vi "Cache.vi"(7 "Action":T1, 8 "error in (no error)":errorcluster, 10 "VI in":variant, 11 "Thread Name":string) -> (0 "error out":errorcluster, 1 "Found?":bool, 2 "VI out":variant, 3 "Generic VI out":refnum<vi>, 5 "Thread Names":string[](array[string]))   [LabVIEW 2018, in "Thread.lvlib"]
uses:
  Thread.lvlib
  Cache Action.ctl
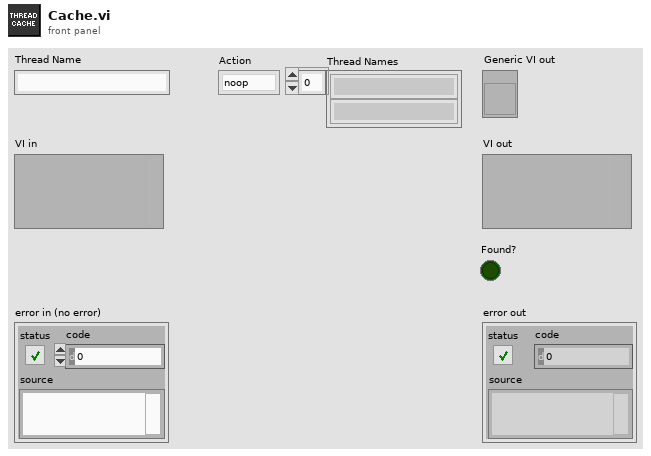
[diagram p1: front panel]
types:
  T1 = typedef "Thread.lvlib/Cache Action.ctl" = enum8{"noop", "get", "add", "remove", "remove_by_ref"}
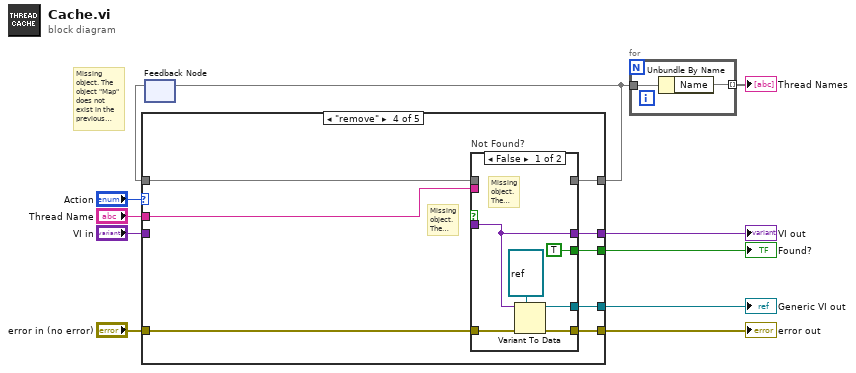
[diagram p0: block diagram]
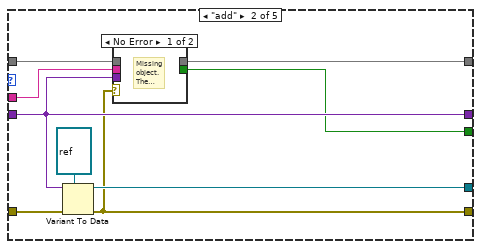
[diagram p3: hidden frame]
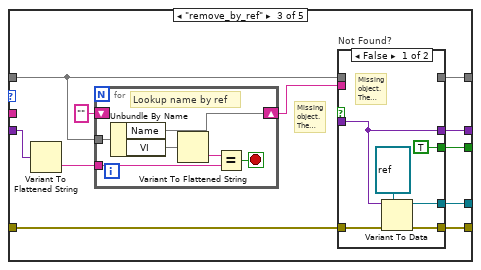
[diagram p5: hidden frame]
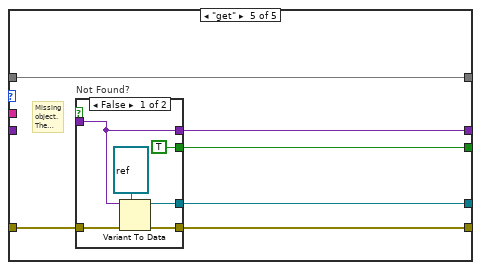
[diagram p8: hidden frame]
diagram:
  # "Missing object. The object \"Map\" does not exist in the previous version."
  n1 = feedback #1() -> (w8, w12)
  n2 = case shown="\"remove\"" "Action" {
    tunnel: [w13 w15 w34 w57 w72] -> w9
    tunnel: "error in (no error)" -> [w13 w23 w35 w58 w73]
    tunnel: [w14 w21 w32 w55 w68] -> w3
    tunnel: w8 -> [w14 w22 w28 w52 w68]
    tunnel: "Thread Name" -> [_ w20 _ w51 _]
    tunnel: "VI in" -> [_ w19 w29 _ _]
    tunnel: [_ w19 w31 w54 w70] -> w5
    tunnel: [_ w17 w33 w56 w71] -> w4
    tunnel: [_ w16 w30 w53 w69] -> w1
    frame "noop" {
    }
    frame "add" {
      n3 = Variant To Data(error in=w23, type=refnum<vi> refnum ("Generic VI out"), Variant=w19) -> (data=w17:refnum<vi>, error out=w15:errorcluster)
      n4 = case shown="No Error" w15 {
        tunnel: w22 -> [_ w24]
        tunnel: [_ w24] -> w21
        tunnel: w20 -> [_ _]
        tunnel: w19 -> [_ _]
        tunnel: [_ _] -> w16
        frame No Error {
          # "Missing object. The object \"Insert Into Map\" does not exist in the previous version."
        }
        frame Error {
        }
      }
    }
    frame "remove_by_ref" {
      # "Missing object. The object \"Look In Map\" does not exist in the previous version."
      n5 = Variant To Flattened String(Variant=w29) -> (data string=w26:string)  [unwired: 1 out]
      n6 = for {
        tunnel: w28 -> [w41]
        shift-right: [w39] -> w25
        shift-left: "" ("Name") -> [_]
        tunnel: w26 -> [w37]
        stop <- w36 stop-if-true
        # "Lookup name by ref"
        n7 = Unbundle By Name(w41) -> ("Name"=w39, "VI"=w40)
        n8 = Variant To Flattened String(Variant=w40) -> (data string=w38:string)  [unwired: 1 out]
        n9 = Equal?(x=w38, y=w37) -> (x = y?=w36:bool)
      }
      n10 = case "Not Found?" shown="False" {
        selector: _ -> [_ _]
        tunnel: w35 -> [w48 w49]
        tunnel: [w47 w49] -> w34
        tunnel: [w45 _] -> w33
        tunnel: w28 -> [_ w50]
        tunnel: [w44 w50] -> w32
        tunnel: w25 -> [_ _]
        tunnel: _ -> [w43 _]
        tunnel: [w43 _] -> w31
        tunnel: [TRUE _] -> w30
        frame False {
          # "Missing object. The object \"Remove From Map\" does not exist in the previous version."
          n11 = Variant To Data(error in=w48, type=refnum<vi> refnum ("Generic VI out"), Variant=w43) -> (data=w45:refnum<vi>, error out=w47:errorcluster)
        }
        frame True {
        }
      }
    }
    frame "remove" {
      # "Missing object. The object \"Look In Map\" does not exist in the previous version."
      n12 = case "Not Found?" shown="False" {
        selector: _ -> [_ _]
        tunnel: w58 -> [w65 w66]
        tunnel: [w64 w66] -> w57
        tunnel: [w62 _] -> w56
        tunnel: w52 -> [_ w67]
        tunnel: [w61 w67] -> w55
        tunnel: w51 -> [_ _]
        tunnel: _ -> [w60 _]
        tunnel: [w60 _] -> w54
        tunnel: [TRUE _] -> w53
        frame False {
          # "Missing object. The object \"Remove From Map\" does not exist in the previous version."
          n13 = Variant To Data(error in=w65, type=refnum<vi> refnum ("Generic VI out"), Variant=w60) -> (data=w62:refnum<vi>, error out=w64:errorcluster)
        }
        frame True {
        }
      }
    }
    frame "get" {
      # "Missing object. The object \"Look In Map\" does not exist in the previous version."
      n14 = case "Not Found?" shown="False" {
        selector: _ -> [_ _]
        tunnel: w73 -> [w79 w80]
        tunnel: [w78 w80] -> w72
        tunnel: [w76 _] -> w71
        tunnel: _ -> [w75 _]
        tunnel: [w75 _] -> w70
        tunnel: [TRUE _] -> w69
        frame False {
          n15 = Variant To Data(error in=w79, type=refnum<vi> refnum ("Generic VI out"), Variant=w75) -> (data=w76:refnum<vi>, error out=w78:errorcluster)
        }
        frame True {
        }
      }
    }
  }
  "error out" <- w9
  "Generic VI out" <- w4
  "VI out" <- w5
  "Found?" <- w1
  n16 = feedback-in #1(w3) -> ()
  n17 = for {
    tunnel: w3 -> [w82]
    tunnel: [w81] -> w2 mode=indexing
    n18 = Unbundle By Name(w82) -> ("Name"=w81)
  }
  "Thread Names" <- w2
